vi "AddCircle.vi"(4 "centerY":dbl, 6 "centerX":dbl, 9 "radius":dbl=34.0, 10 "vertical":dbl[](array[numeric]), 11 "horizontal":dbl[](array[numeric])) -> (3 "output":cluster{"horizontal":dbl[], "vertical":dbl[]}[](array[cluster]))   [LabVIEW 2012]
panel:
  out "x":dbl[](array[numeric])
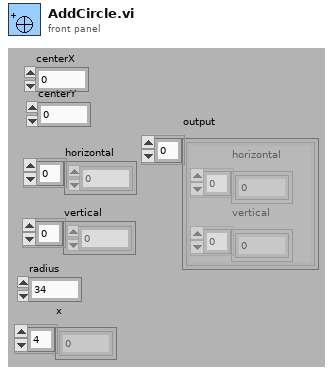
[diagram p1: front panel]
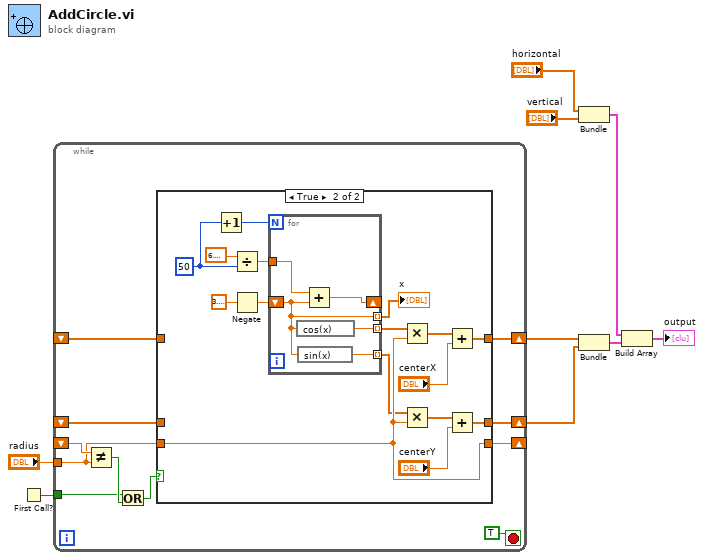
[diagram p0: block diagram]
diagram:
  n1 = First Call?() -> (First Call?: T/F=w7:bool)
  n2 = while {
    shift-right: [w19] -> w9
    shift-left: _ -> [w17]
    shift-right: [w18] -> w8
    shift-left: _ -> [w16]
    shift-right: [w15] -> _
    shift-left: _ -> [w14]
    tunnel: w7 -> [w11]
    tunnel: "radius" -> [w10]
    stop <- TRUE stop-if-true
    n3 = Not Equal?(x=w14, y=w10) -> (x != y?=w13:bool)
    n4 = Or(x=w11, y=w13) -> (x .or. y?=w12:bool)
    n5 = case shown="True" w12 {
      tunnel: [w23 w35] -> w19
      tunnel: [w22 w34] -> w18
      tunnel: w17 -> [w23 _]
      tunnel: w16 -> [w22 _]
      tunnel: w10 -> [w21 w33]
      tunnel: [w21 w33] -> w15
      frame False {
      }
      frame True {
        w30 = 50
        n6 = Increment(x=w30) -> (x+1=w29:i32)
        n7 = Divide(x=6.283185307179586, y=w30) -> (x/y=w32:dbl)
        n8 = Negate(x=3.141592653589793) -> (-x=w31:dbl)
        n9 = for {
          N: w29 -> [_]
          shift-right: [w43] -> _
          shift-left: w31 -> [w42]
          tunnel: w32 -> [w44]
          tunnel: [w42] -> w24 mode=indexing
          tunnel: [w41] -> w25 mode=indexing
          tunnel: [w40] -> w26 mode=indexing
          n10 = expression code="cos(x)"(w42) -> (w40:dbl)
          n11 = expression code="sin(x)"(w42) -> (w41:dbl)
          n12 = Add(x=w44, y=w42) -> (x+y=w43:dbl)
        }
        "x" <- w24
        n13 = Multiply(x=w26, y=w33) -> (x*y=w39:dbl[])
        n14 = Multiply(x=w25, y=w33) -> (x*y=w38:dbl[])
        n15 = Add(x=w39, y="centerX") -> (x+y=w35:dbl[])
        n16 = Add(x=w38, y="centerY") -> (x+y=w34:dbl[])
      }
    }
  }
  n17 = Bundle("horizontal"="horizontal", "vertical"="vertical") -> (w4:cluster{"horizontal":dbl[], "vertical":dbl[]})  [unwired: 1 in]
  n18 = Bundle(w9, w8) -> (w3:cluster{dbl[], dbl[]})  [unwired: 1 in]
  n19 = Build Array(w4, w3) -> (→"output":cluster{"horizontal":dbl[], "vertical":dbl[]}[])
